vi "检测IP字符串是否有效.vi"(11 "IP地址":string="192.168.1.100") -> (0 "有效IP？":bool)   [LabVIEW 2017]
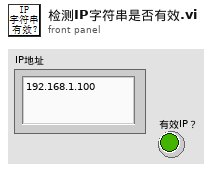
[diagram p1: front panel]
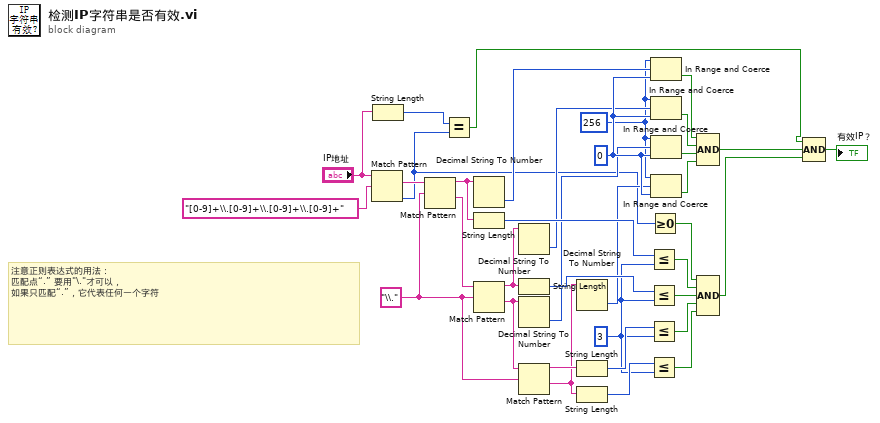
[diagram p0: block diagram]
diagram:
  w17 = 0
  w8 = 256
  w28 = 3 ("y")
  w35 = "\\." ("正则表达式")
  # "注意正则表达式的用法：\n匹配点“.” 要用\"\\.\"才可以，\n如果只匹配“.”，它代表任何一个字符"
  n1 = Match Pattern(string="IP地址", regular expression="[0-9]+\\.[0-9]+\\.[0-9]+\\.[0-9]+" ("正则表达式")) -> (match substring=w36:string, offset past match=w4:i32)  [unwired: 1 in, 2 out]
  n2 = String Length(string="IP地址") -> (length=w2:i32)
  n3 = Match Pattern(string=w36, regular expression=w35) -> (before substring=w21:string, after substring=w34:string)  [unwired: 1 in, 2 out]
  n4 = Equal?(x=w2, y=w4) -> (x = y?=w1:bool)
  n5 = Decimal String To Number(string=w21) -> (number=w20:i32)  [unwired: 2 in, 1 out]
  n6 = String Length(string=w21) -> (length=w32:i32)
  n7 = Match Pattern(string=w34, regular expression=w35) -> (before substring=w16:string, after substring=w10:string)  [unwired: 1 in, 2 out]
  n8 = Decimal String To Number(string=w16) -> (number=w15:i32)  [unwired: 2 in, 1 out]
  n9 = String Length(string=w16) -> (length=w31:i32)
  n10 = Decimal String To Number(string=w10) -> (number=w9:i32)  [unwired: 2 in, 1 out]
  n11 = Match Pattern(string=w10, regular expression=w35) -> (before substring=w33:string, after substring=w7:string)  [unwired: 1 in, 2 out]
  n12 = Decimal String To Number(string=w7) -> (number=w6:i32)  [unwired: 2 in, 1 out]
  n13 = String Length(string=w33) -> (length=w30:i32)
  n14 = String Length(string=w7) -> (length=w29:i32)
  n15 = Less Or Equal?(x=w32, y=w28) -> (x <= y?=w26:bool)
  n16 = Less Or Equal?(x=w31, y=w28) -> (x <= y?=w25:bool)
  n17 = Less Or Equal?(x=w30, y=w28) -> (x <= y?=w24:bool)
  n18 = Less Or Equal?(x=w29, y=w28) -> (x <= y?=w23:bool)
  n19 = Greater Or Equal To 0?(x=w4) -> (x >= 0?=w27:bool)
  n20 = In Range and Coerce(upper limit=w8, x=w20, lower limit=w17) -> (In Range?=w18:bool)  [unwired: 1 out]
  n21 = In Range and Coerce(upper limit=w8, x=w15, lower limit=w17) -> (In Range?=w14:bool)  [unwired: 1 out]
  n22 = In Range and Coerce(upper limit=w8, x=w9, lower limit=w17) -> (In Range?=w13:bool)  [unwired: 1 out]
  n23 = In Range and Coerce(upper limit=w8, x=w6, lower limit=w17) -> (In Range?=w12:bool)  [unwired: 1 out]
  n24 = Compound Arithmetic op=AND(w18, w14, w13, w12) -> (w11:bool)
  n25 = Compound Arithmetic op=AND(w27, w26, w25, w24, w23) -> (w22:bool)
  n26 = Compound Arithmetic op=AND ("复合运算")(w1, w11, w22) -> (→"有效IP？":bool)
